vi "Drift Data to file (SubVI).vi"(6 "z drift":dbl, 8 "Comment":string, 9 "y Drift":sgl, 10 "X drift":sgl, 11 "Byte Stream File in":refnum<file>) -> (3 "Byte Stream File out":refnum<file>)   [LabVIEW 2014]
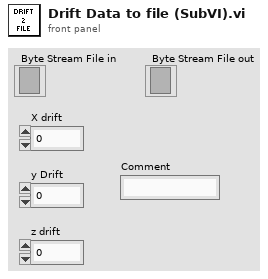
[diagram p1: front panel]
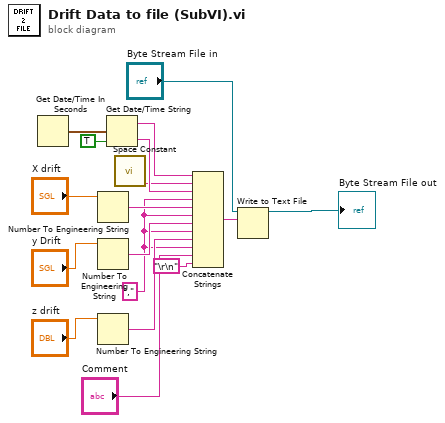
[diagram p0: block diagram]
diagram:
  w2 = "," ("string")
  n1 = Get Date/Time In Seconds() -> (seconds since 1Jan1904=w13:timestamp)
  n2 = Number To Engineering String(4:"X drift") -> (0:w10:string)  [unwired: 3 in]
  n3 = Number To Engineering String(4:"y Drift") -> (0:w15:string)  [unwired: 3 in]
  n4 = Number To Engineering String(4:"z drift") -> (0:w16:string)  [unwired: 3 in]
  n5 = Get Date/Time String(seconds (now)=w13, want seconds? (F)=TRUE) -> (date string=w5:string, time string=w14:string)  [unwired: 1 in]
  n6 = call <vilib>:"Space Constant.vi"() -> ("String"=w4:string)
  n7 = Concatenate Strings(w5, w4, w14, w2, w10, w2, w15, w2, w16, w2, "Comment", "\r\n") -> (w8:string)
  n8 = Write to Text File(file (use dialog)="Byte Stream File in", text=w8) -> (refnum out=→"Byte Stream File out":refnum<file>)  [unwired: 2 in, 2 out]
